vi "save channels to interleaved multi-tiff files.vi"(8 "frame number in":i32, 9 "last frame":bool, 11 "image data in":dbl[][](array[numeric])) -> ()   [LabVIEW 2012]
uses:
  Custom Controls/file format type def.ctl
  GFG/GFGpathGet.vi
  GFG/GFGnumericGet.vi
  Libtiff3/libtiff3.llb/libtiff3.lvlib
  GFG/GFG library.lvlib
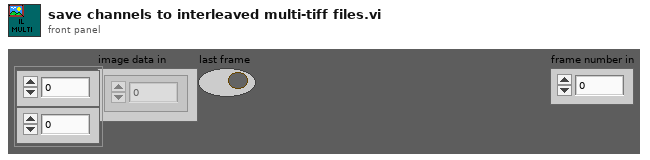
[diagram p1: front panel]
types:
  T1 = typedef "file format type def.ctl" = enum16{"16bit raw", "32bit raw", "16bit multi-tiff (interleave)", "16bit multi-tiff (separate)", "16bit multi-tiff (stacked)", "32bit multi-tiff (interleave)", "32bit multi-tiff (separate)", "32bit multi-tiff (stacked)", "16bit tiff series (interleave)", "16bit tiff series (separate)", "16bit tiff series (stacked)", "32bit tiff series (interleave)", "32bit tiff series (separate)", "32bit tiff series (stacked)"}
  T2 = cluster{"no..of.frames.to.acquire":dbl, "x.pixels":dbl, "y.pixels":dbl, "x.pixel.sz":dbl, "y.pixel.sz":dbl}
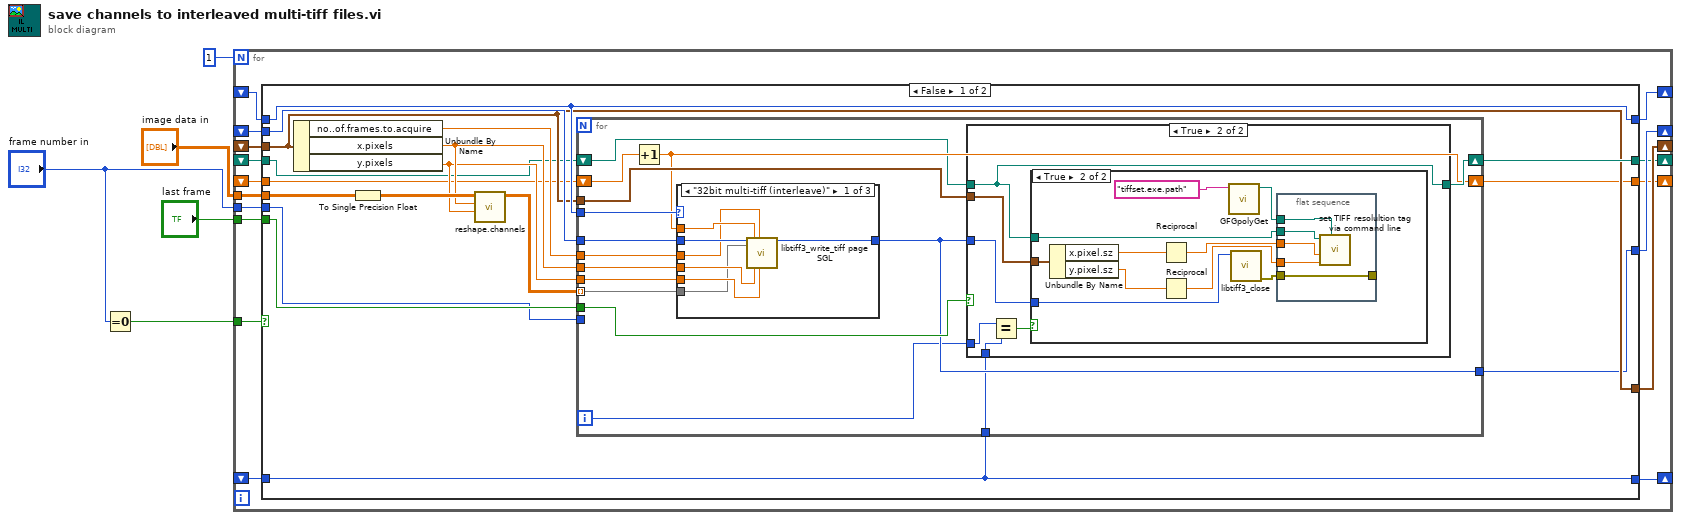
[diagram p0: block diagram]
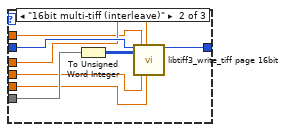
[diagram p2: hidden frame]
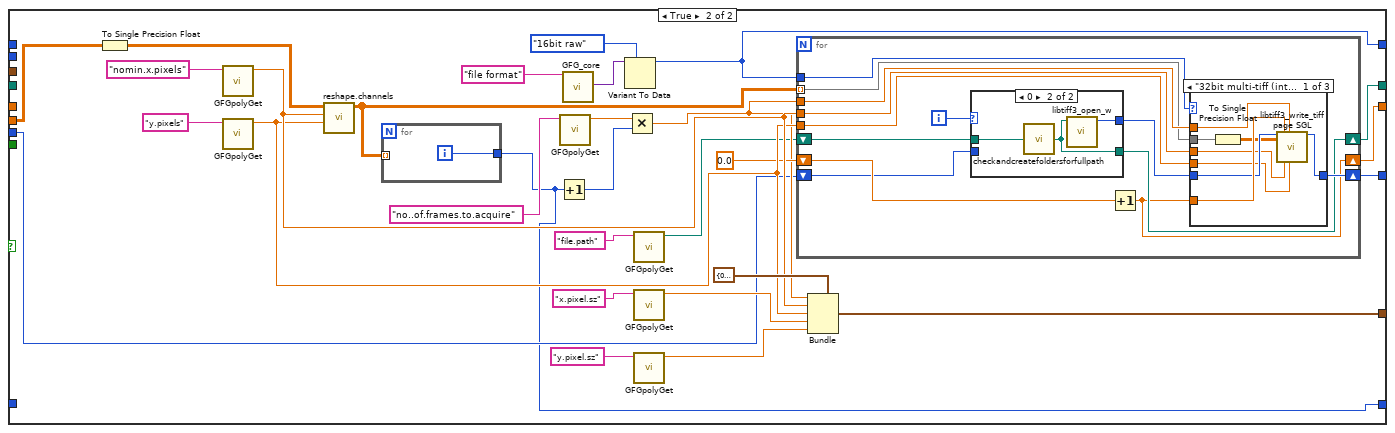
[diagram p6: hidden frame]
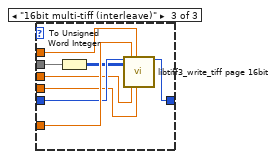
[diagram p9: hidden frame]
diagram:
  n1 = Equal To 0?(x="frame number in") -> (x = 0?=w4:bool)
  n2 = for {
    N: 1 -> [_]
    tunnel: w4 -> [w21]
    shift-right: [w20] -> _
    shift-left: _ -> [w19]
    tunnel: "image data in" -> [w18]
    shift-right: [w17] -> _
    shift-left: _ -> [w16]
    shift-right: [w15] -> _
    shift-left: _ -> [w14]
    shift-right: [w13] -> _
    shift-left: _ -> [w12]
    tunnel: "last frame" -> [w11]
    tunnel: "frame number in" -> [w10]
    shift-right: [w9] -> _
    shift-left: _ -> [w8]
    shift-right: [w7] -> _
    shift-left: _ -> [w6]
    n3 = case shown="False" w21 {
      tunnel: w16 -> [w33 _]
      tunnel: [w31 w105] -> w20
      tunnel: w19 -> [w37 _]
      tunnel: w18 -> [w30 w101]
      tunnel: [w33 w107] -> w17
      tunnel: [w32 w108] -> w15
      tunnel: w14 -> [w32 _]
      tunnel: [w36 w100] -> w13
      tunnel: w12 -> [w23 _]
      tunnel: w11 -> [w38 _]
      tunnel: w10 -> [w34 w95]
      tunnel: [w24 w98] -> w9
      tunnel: w8 -> [w25 _]
      tunnel: [w22 w92] -> w7
      tunnel: w6 -> [w22 _]
      frame False {
        n4 = Unbundle By Name(w32) -> ("no..of.frames.to.acquire"=w35:dbl, "x.pixels"=w27:dbl, "y.pixels"=w26:dbl)
        n5 = To Single Precision Float(number=w30) -> (single precision float=w29:sgl[][])
        n6 = call "reshape.channels.vi"("y.pixels"=w26, "x.pixels"=w27, "element"=w29) -> ("Array"=w28:dbl[][][])  [unwired: 8 in]
        n7 = for {
          tunnel: w38 -> [w53]
          tunnel: w28 -> [w52] mode=indexing
          tunnel: w37 -> [w51]
          tunnel: w35 -> [w49]
          tunnel: w34 -> [_]
          tunnel: w27 -> [w48]
          tunnel: w26 -> [w47]
          tunnel: w33 -> [w46]
          tunnel: w32 -> [w45]
          tunnel: [w44] -> w31
          shift-right: [w42] -> w24
          shift-left: w25 -> [w43]
          shift-right: [w50] -> w36
          shift-left: w23 -> [w41]
          tunnel: w22 -> [w40]
          i -> [w39]
          n8 = Increment(x=w43) -> (x+1=w42:dbl)
          n9 = case shown="\"32bit multi-tiff (interleave)\"" w46 {
            tunnel: w52 -> [w54 w68 _]
            tunnel: w51 -> [w60 w66 w69]
            tunnel: [w57 w65 w69] -> w44
            tunnel: w49 -> [w58 w64 _]
            tunnel: w42 -> [w59 w63 _]
            tunnel: w48 -> [w56 w62 _]
            tunnel: w47 -> [w55 w61 _]
            frame "32bit multi-tiff (interleave)" {
              n10 = call "libtiff3_write_tiff page SGL.vi"("Handle"=w60, "Image Pixels (Float)"=w54, "page"=w59, "x.pixels"=w56, "totalpages"=w58, "y.pixels"=w55) -> ("Handle out"=w57:i32)  [unwired: 12 in, 1 out]
            }
            frame "16bit multi-tiff (interleave)" {
              n11 = To Unsigned Word Integer(number=w68) -> (unsigned 16bit integer=w67:u16[][])
              n12 = call "libtiff3_write_tiff page 16bit.vi"("Handle"=w66, "Image Pixels (U16)"=w67, "page"=w63, "x.pixels"=w62, "totalpages"=w64, "y.pixels"=w61) -> ("Handle out"=w65:i32)  [unwired: 12 in, 1 out]
            }
            frame Default {
            }
          }
          n13 = case shown="True" w53 {
            tunnel: w45 -> [_ w76]
            tunnel: w41 -> [w70 w71]
            tunnel: w44 -> [_ w75]
            tunnel: [w70 w71] -> w50
            tunnel: w40 -> [_ w72]
            tunnel: w39 -> [_ w73]
            frame False {
            }
            frame True {
              n14 = Equal?(x=w73, y=w72) -> (x = y?=w74:bool)
              n15 = case shown="True" w74 {
                tunnel: w76 -> [_ w81]
                tunnel: w71 -> [_ w80]
                tunnel: w75 -> [_ w79]
                frame False {
                }
                frame True {
                  n16 = Unbundle By Name(w81) -> ("x.pixel.sz"=w82:dbl, "y.pixel.sz"=w83:dbl)
                  n17 = Reciprocal(x=w82) -> (1/x=w84:dbl)
                  n18 = Reciprocal(x=w83) -> (1/x=w85:dbl)
                  n19 = call-poly "GFGpolyGet.vi"("Variable Name in"="tiffset.exe.path") -> ("Path"=w77:path)  [unwired: 9 in, 1 out]
                  n20 = call "libtiff3_close.vi"("Handle"=w79) -> ("error out"=w86:errorcluster)  [unwired: 9 in]
                  n21 = flat-sequence {
                    tunnel: w80 -> [w91]
                    tunnel: w86 -> [w88]
                    tunnel: w84 -> [w90]
                    tunnel: w85 -> [w89]
                    tunnel: [w88] -> _
                    tunnel: w77 -> [w87]
                    frame #0 {
                      n22 = call "set TIFF resolultion tag via command line.vi"("tiffset.exe file path"=w87, "y pixels per m"=w89, "x pixels per m"=w90, "TIFF file path"=w91) -> ()  [unwired: 8 in]
                    }
                  }
                }
              }
            }
          }
        }
      }
      frame True {
        n23 = To Single Precision Float(number=w101) -> (single precision float=w104:sgl[][])
        n24 = call-poly "GFGpolyGet.vi"("Variable Name in"="nomin.x.pixels" ("Tag in")) -> ("Numeric"=w103:dbl)  [unwired: 9 in, 1 out]
        n25 = call-poly "GFGpolyGet.vi"("Variable Name in"="y.pixels" ("Tag in")) -> ("Numeric"=w102:dbl)  [unwired: 9 in, 1 out]
        n26 = call "reshape.channels.vi"("y.pixels"=w102, "x.pixels"=w103, "element"=w104) -> ("Array"=w97:dbl[][][])  [unwired: 8 in]
        n27 = for {
          tunnel: w97 -> [_] mode=indexing
          tunnel: [w121] -> w92
          i -> [w121]
        }
        n28 = Increment(x=w92) -> (x+1=w93:i32)
        n29 = call-poly "GFGpolyGet.vi"("Variable Name in"="no..of.frames.to.acquire") -> ("Numeric"=w106:dbl)  [unwired: 9 in, 1 out]
        n30 = call "GFG_core.vi"("Variable Name in"="file format") -> ("Variant Out"=w119:variant)  [unwired: 12 in, 6 out]
        n31 = Variant To Data(type=file_format_type_def."16bit raw" ("file format"), Variant=w119) -> (data=w107:T1)  [unwired: 1 in, 1 out]
        n32 = Multiply(x=w106, y=w93) -> (x*y=w96:dbl)
        n33 = call-poly "GFGpolyGet.vi"("Variable Name in"="file.path") -> ("Path"=w94:path)  [unwired: 9 in, 1 out]
        n34 = call-poly "GFGpolyGet.vi"("Variable Name in"="x.pixel.sz" ("Tag in")) -> ("Numeric"=w111:dbl)  [unwired: 9 in, 1 out]
        n35 = call-poly "GFGpolyGet.vi"("Variable Name in"="y.pixel.sz" ("Tag in")) -> ("Numeric"=w110:dbl)  [unwired: 9 in, 1 out]
        n36 = for {
          tunnel: w107 -> [w134]
          tunnel: w96 -> [w133]
          tunnel: w103 -> [w131]
          tunnel: w102 -> [w130]
          tunnel: w97 -> [w129] mode=indexing
          shift-right: [w125] -> w98
          shift-left: 0.0 -> [w126]
          shift-right: [w132] -> w105
          shift-left: w95 -> [w123]
          shift-right: [w127] -> w100
          shift-left: w94 -> [w122]
          i -> [w124]
          n37 = case shown="0" w124 {
            tunnel: [w135 w139] -> w128
            tunnel: [w136 w138] -> w127
            tunnel: w122 -> [w136 w137]
            tunnel: w123 -> [w135 _]
            frame 1, Default {
            }
            frame 0 {
              n38 = call "checkandcreatefoldersforfullpath.vi"("Path IN"=w137) -> ("Path OUT"=w138:path)  [unwired: 4 in]
              n39 = call "libtiff3_open_w.vi"("Input path"=w138) -> ("handle"=w139:i32)  [unwired: 9 in, 1 out]
            }
          }
          n40 = Increment(x=w126) -> (x+1=w125:dbl)
          n41 = case shown="\"32bit multi-tiff (interleave)\"" w134 {
            tunnel: w129 -> [w143 _ w153]
            tunnel: w128 -> [w144 w148 w154]
            tunnel: w125 -> [w145 _ w155]
            tunnel: w133 -> [w146 _ w156]
            tunnel: [w147 w148 w149] -> w132
            tunnel: w131 -> [w140 _ w151]
            tunnel: w130 -> [w141 _ w150]
            frame "32bit multi-tiff (interleave)" {
              n42 = To Single Precision Float(number=w143) -> (single precision float=w142:sgl[][])
              n43 = call "libtiff3_write_tiff page SGL.vi"("Handle"=w144, "Image Pixels (Float)"=w142, "page"=w145, "x.pixels"=w140, "totalpages"=w146, "y.pixels"=w141) -> ("Handle out"=w147:i32)  [unwired: 12 in, 1 out]
            }
            frame Default {
            }
            frame "16bit multi-tiff (interleave)" {
              n44 = To Unsigned Word Integer(number=w153) -> (unsigned 16bit integer=w152:u16[][])
              n45 = call "libtiff3_write_tiff page 16bit.vi"("Handle"=w154, "Image Pixels (U16)"=w152, "page"=w155, "x.pixels"=w151, "totalpages"=w156, "y.pixels"=w150) -> ("Handle out"=w149:i32)  [unwired: 12 in, 1 out]
            }
          }
        }
        n46 = Bundle(cluster=T2 {"no..of.frames.to.acquire"=0.0, "x.pixels"=0.0, "y.pixels"=0.0, "x.pixel.sz"=0.0, "y.pixel.sz"=0.0} ("output cluster"), "no..of.frames.to.acquire"=w96, "x.pixels"=w103, "y.pixels"=w102, "x.pixel.sz"=w111, "y.pixel.sz"=w110) -> (w108:T2)
      }
    }
  }
